vi "getPoints.vi"(0 "reference":refnum<class "NoteEdge.lvclass">, 5 "error in (no error)":errorcluster) -> (14 "reference out":refnum<class "NoteEdge.lvclass">, 15 "points":T1[](array[typedef]) {"y" format="%.2f"; "x" format="%.2f"}, 19 "error out":errorcluster)   [LabVIEW 2012, in "NoteEdge.lvclass"]
doc: "getPoints()"
uses:
  <resource>/Framework/Providers/Open_GDS/UML/NoteEdge_class/NoteEdge.lvclass
  <resource>/Framework/Providers/Open_GDS/UML/General/Point/Point Point2D.ctl
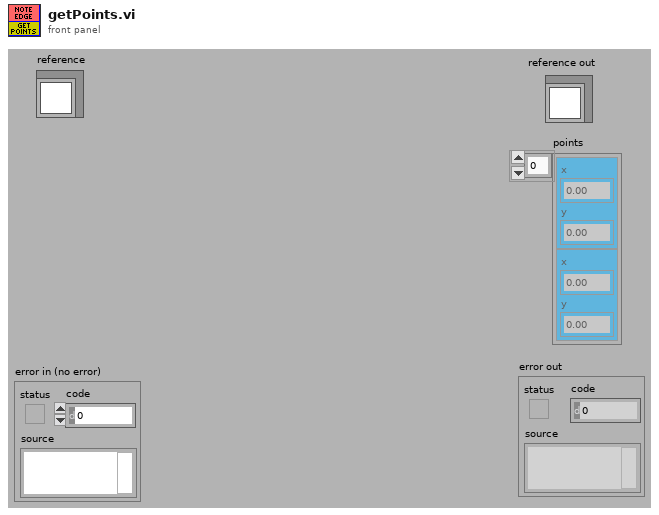
[diagram p1: front panel]
types:
  T1 = typedef "Point Point2D.ctl" = cluster{"x":dbl, "y":dbl}
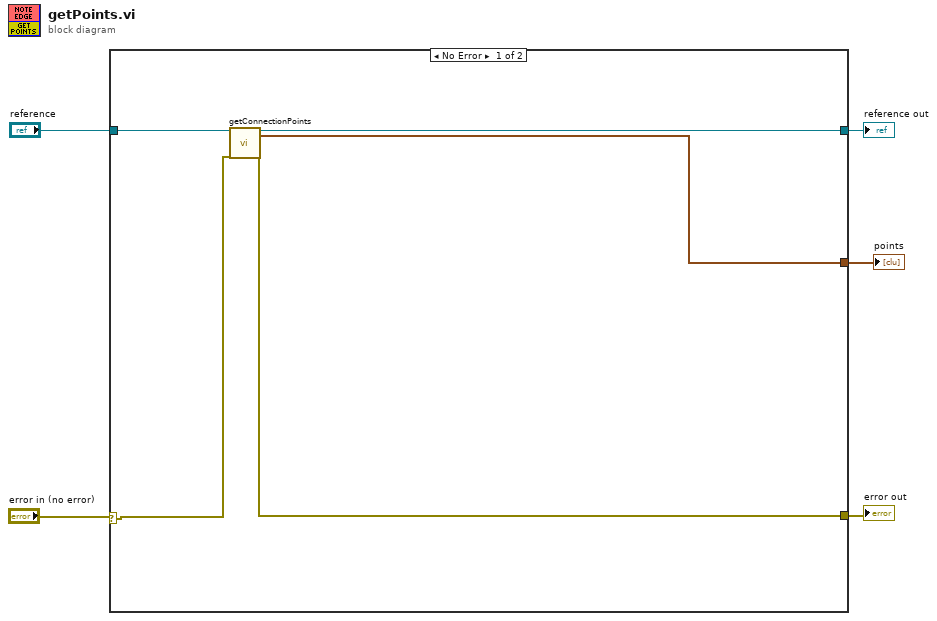
[diagram p0: block diagram]
diagram:
  n1 = case shown="No Error" "error in (no error)" {
    selector: "error in (no error)" -> [w6 w11]
    tunnel: "reference" -> [w10 w12]
    tunnel: [w9 w11] -> w4
    tunnel: [w8 w12] -> w3
    tunnel: [w7 _] -> w1
    frame No Error {
      n2 = call-dynamic "getConnectionPoints.vi"("reference"=w10, "error in (no error)"=w6) -> ("reference out"=w8:refnum<class "NoteEdge.lvclass">, "connectionPoints"=w7:T1[], "error out"=w9:errorcluster)  [unwired: 15 in]
    }
    frame Error {
    }
  }
  "reference out" <- w3
  "error out" <- w4
  "points" <- w1
